vi "S7Com_TPKT_READ(SubVI).vi"(4 "error in":errorcluster, 5 "timeout ms (25000)":i32, 7 "connection ID in":refnum<k5>) -> (0 "error out":errorcluster, 1 "TPDU Data":T1 format="X%02x", 2 "Hdr Error":bool, 3 "connection ID out":refnum<k5>)   [LabVIEW 2018]
doc: "Reads the Transport Packt (TPKT) and outputs the Transport Data Unit (TDU)."
uses:
  S7Com_HexByteArray.ctl
  S7Com_HexByte.ctl
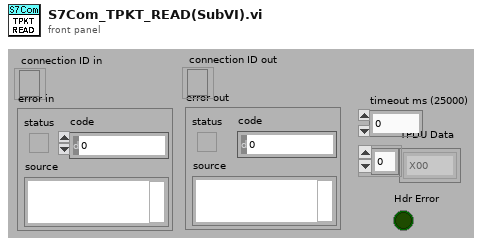
[diagram p1: front panel]
types:
  T1 = typedef "S7Com_HexByteArray.ctl" = T2[]
  T2 = typedef "S7Com_HexByte.ctl" = u8
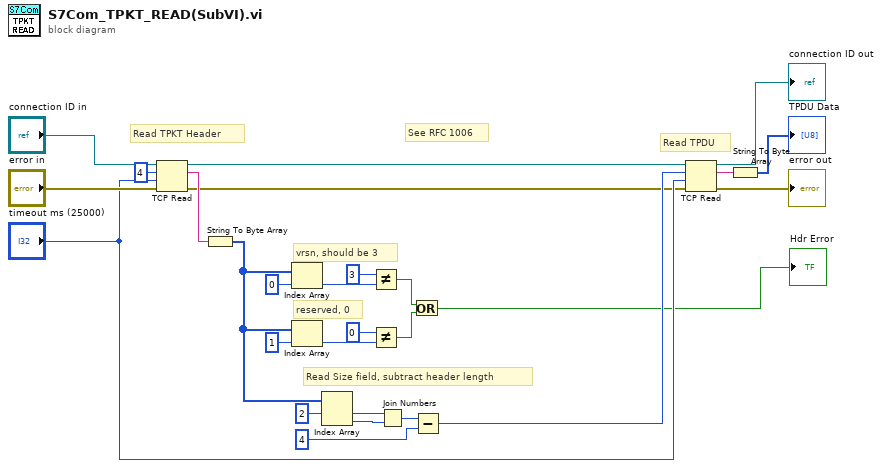
[diagram p0: block diagram]
diagram:
  # "See RFC 1006"
  # "reserved, 0"
  # "vrsn, should be 3"
  # "Read Size field, subtract header length"
  # "Read TPDU"
  # "Read TPKT Header"
  n1 = TCP Read(connection ID="connection ID in", bytes to read=4, error in (no error)="error in", 9:"timeout ms (25000)") -> (connection ID out=w21:refnum<k5>, data out=w27:string, error out=w1:errorcluster)  [unwired: 1 out]
  n2 = String To Byte Array(string=w27) -> (unsigned byte array=w10:u8[])
  n3 = Index Array(array=w10, index=0) -> (element=w8:u8)
  n4 = Index Array(array=w10, index=1) -> (element=w5:u8)
  n5 = Index Array(array=w10, index #1=2) -> (element #1=w15:u8, element #2=w16:u8)  [unwired: 1 in]
  n6 = Not Equal?(x=u8 3, y=w8) -> (x != y?=w4:bool)
  n7 = Not Equal?(x=u8 0, y=w5) -> (x != y?=w3:bool)
  n8 = Join Numbers(hi=w15, lo=w16) -> ((hi.lo)=w17:u16)
  n9 = Or(x=w4, y=w3) -> (x .or. y?=→"Hdr Error":bool)
  n10 = Subtract(x=w17, y=u16 4) -> (x-y=w9:u16)
  n11 = TCP Read(connection ID=w21, bytes to read=w9, error in (no error)=w1, 9:"timeout ms (25000)") -> (connection ID out=→"connection ID out":refnum<k5>, data out=w25:string, error out=→"error out":errorcluster)  [unwired: 1 out]
  n12 = String To Byte Array(string=w25) -> (unsigned byte array=→"TPDU Data":u8[])
